vi "Log In.vi"() -> (1 "Logged":bool, 2 "user type":string, 3 "username":string)   [LabVIEW 2014]
doc: "This VI is used to login user and check for user credentials\nif ok it returns username and type (norma/admin) else it returns NULL"
uses:
  <vilib>/addons/database/_DB Variant To Data/Database Variant To Data.xnode
panel:
  # "Outputs"
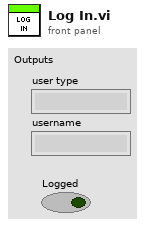
[diagram p1: front panel]
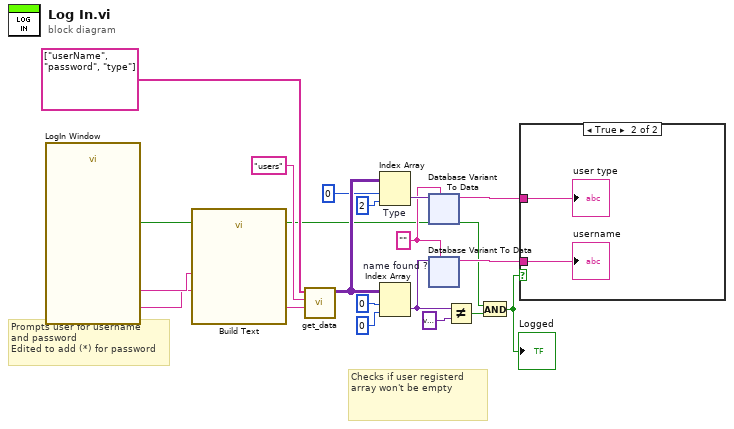
[diagram p0: block diagram]
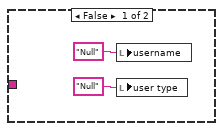
[diagram p2: hidden frame]
diagram:
  w4 = "" ("table")
  # "Checks if user registerd array won't be empty"
  # "Prompts user for username\nand password\nEdited to add (*) for password"
  n1 = call "LogIn Window.vi"() -> ("Password"=w14:string, "Username"=w15:string, "OK"=w2:bool)  [unwired: 16 in, 1 out]
  n2 = call "Build Text"("username"=w15, "password"=w14) -> ("Result"=w13:string)  [unwired: 12 in, 1 out]
  n3 = call "get_data.vi"("condition"=w13, "table"="users", "columns"=string[] ["userName", "password", "type"]) -> ("Data"=w9:variant[][])  [unwired: 5 in, 3 out]
  n4 = Index Array "Type"(array=w9, index (row)=0, index (col)=2 ("disabled index (col)")) -> (element=w5:variant)
  n5 = Index Array "name found ?"(array=w9, index (row)=0, index (col)=0 ("disabled index (col)")) -> (element=w6:variant)
  n6 = xnode "Database Variant To Data"("database variant"=w5, "type"=w4) -> ("data"=w19:string)  [unwired: 1 in, 1 out]
  n7 = xnode "Database Variant To Data"("database variant"=w6, "type"=w4) -> ("data"=w18:string)  [unwired: 1 in, 1 out]
  n8 = Not Equal?(x=w6, y=variant) -> (x != y?=w3:bool)
  n9 = And(x=w2, y=w3) -> (x .and. y?=w1:bool)
  "Logged" <- w1
  n10 = case shown="True" w1 {
    tunnel: w19 -> [_ w23]
    tunnel: w18 -> [_ w22]
    frame False {
      n11 = local write "username"("Null" ("user type")) -> ()
      n12 = local write "user type"("Null" ("user type")) -> ()
    }
    frame True {
      "user type" <- w23
      "username" <- w22
    }
  }
